vi "Router - Handshaking Test.vi"() -> ()   [LabVIEW 2016]
uses:
  <vilib>/pximc/Initialize Reader Session (U32).vi
  <vilib>/pximc/Connect (U32).vi
  <vilib>/pximc/Read (U32).vi
  PXImc Router.lvlib
  <vilib>/pximc/nipximc.lvlib
panel:
  in  "Connection Timeout (s)":dbl
  out "Data Out 2":u32[](array[numeric])
  in  "Resource Name In":string
  in  "Reader Buffer Size In":u64
  in  "Reader Conn ID":u16
  in  "# Elements to Read":i32
  out "error out":errorcluster
  out "Data Out":u32[](array[numeric])
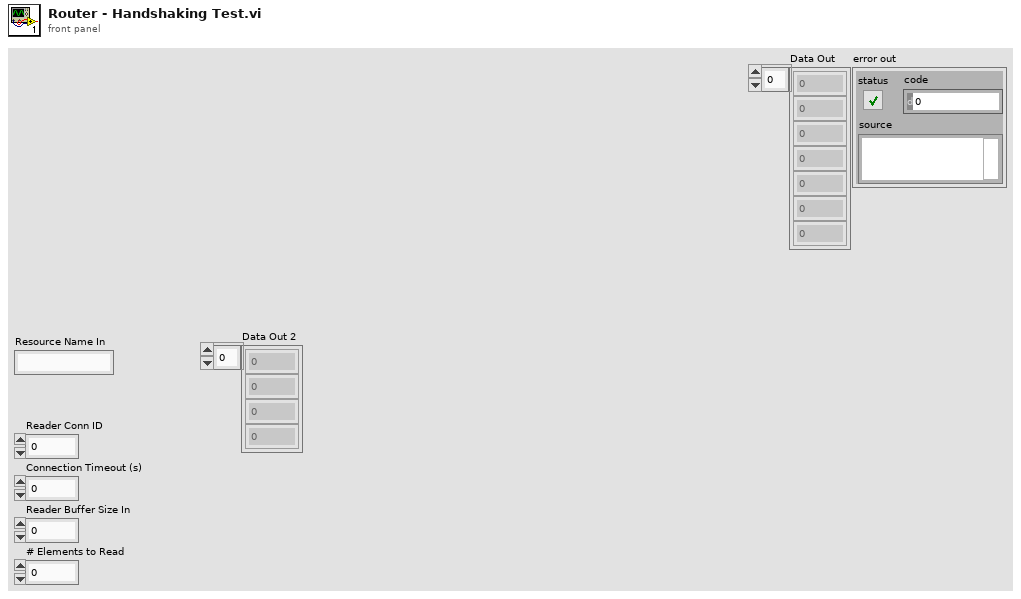
[diagram p1: front panel]
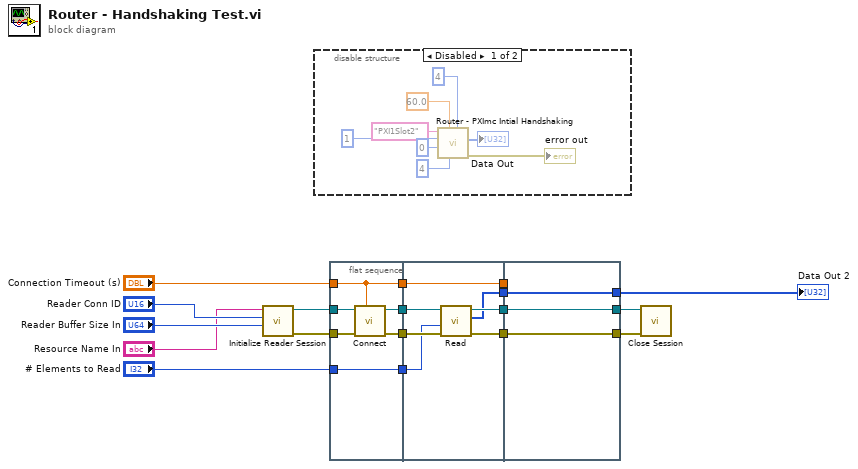
[diagram p0: block diagram]
diagram:
  n1 = call-poly <vilib>:"Initialize Reader Session.vi"("buffer size"="Reader Buffer Size In", "writer's connection id (1)"="Reader Conn ID", "interface"="Resource Name In") -> ("error out"=w2:errorcluster, "session out"=w1:refnum<k21>)  [unwired: 7 in]
  n2 = disable-structure shown="Disabled" {
    frame Disabled {
      n3 = call "Router - PXImc Intial Handshaking.vi"("Reader Buffer Size In"=u64 4, "# Elements to Read"=4, "Connection Timeout (s)"=60.0, "Reader Conn ID"=u16 0, "Writer Conn ID"=u16 1, "Resource Name In"="PXI1Slot2") -> ("error out"=→"error out":errorcluster, "Data Out"=→"Data Out":u32[])  [unwired: 4 in]
    }
    frame Enabled {
    }
  }
  n4 = flat-sequence {
    tunnel: w1 -> [w32]
    tunnel: w2 -> [w31]
    tunnel: [w30] -> w12
    tunnel: [w29] -> w11
    tunnel: "Connection Timeout (s)" -> [w27]
    tunnel: "# Elements to Read" -> [w28]
    tunnel: [w28] -> w10
    tunnel: [w27] -> w9
    tunnel: w12 -> [w39]
    tunnel: w11 -> [w37]
    tunnel: [w38] -> w8
    tunnel: [w36] -> w7
    tunnel: [w35] -> w6
    tunnel: w10 -> [w34]
    tunnel: w9 -> [w33]
    tunnel: [w33] -> w5
    tunnel: [w41] -> w4
    tunnel: [w42] -> w3
    tunnel: w8 -> [w42]
    tunnel: w7 -> [w41]
    tunnel: w6 -> [w40]
    tunnel: [w40] -> w14
    tunnel: w5 -> [_]
    frame #0 {
      n5 = call-poly <vilib>:"Connect.vi"("timeout in seconds (-1)"=w27, "error in (no error)"=w31, "session in"=w32) -> ("error out"=w29:errorcluster, "session out"=w30:refnum<k21>)  [unwired: 7 in]
    }
    frame #1 {
      n6 = call-poly <vilib>:"Read.vi"("error in (no error)"=w37, "number of elements"=w34, "session in"=w39) -> ("error out"=w36:errorcluster, "data"=w35:u32[], "session out"=w38:refnum<k21>)  [unwired: 6 in]
    }
    frame #2 {
    }
  }
  n7 = call <vilib>:"Close Session.vi"("error in (no error)"=w4, "session in"=w3) -> ()  [unwired: 9 in, 1 out]
  "Data Out 2" <- w14
